vi "main_joystick_test.vi"() -> ()   [LabVIEW 2009]
uses:
  <vilib>/Utility/inputDevices.llb/joystickAcquire.vi
  <vilib>/Utility/inputDevices.llb/closeJoystick.vi
panel:
  out "joystick info":T1(array[cluster]) caption="Angaben zum Joystick"
  out "button 4":bool
  out "button 3":bool
  out "button 2":bool
  out "button 1":bool
  in  "Stopp":bool
  out "error out":errorcluster
  out "Joystick ID":refnum<k1> caption="Geräte-ID"
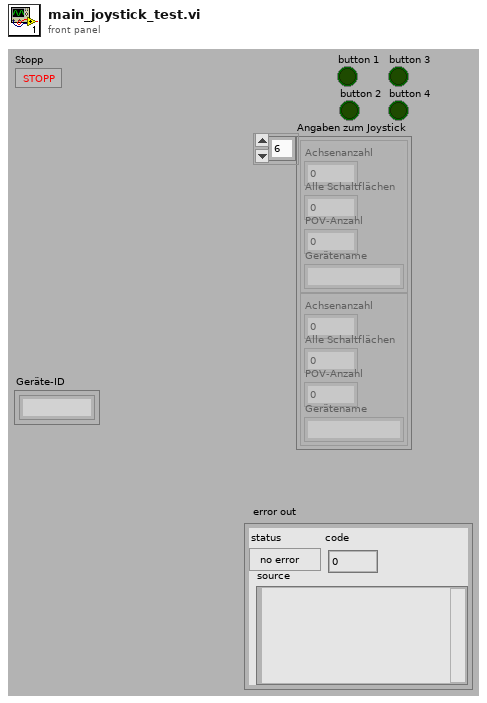
[diagram p1: front panel]
types:
  T1 = cluster{"axes total":u32, "buttons total":u32, "pov total":u32, "device name":string}[]
  T2 = cluster{"X axis":i32, "Y axis":i32, "Z axis":i32, "X axis rotation":i32, "Y axis rotation":i32, "Z axis rotation":i32, "U axis":i32, "V axis":i32}
  T3 = cluster{"button 1":bool, "button 2":bool, "button 3":bool, "button 4":bool, "button 5":bool, "button 6":bool, "button 7":bool, "button 8":bool, "button 9":bool, "button 10":bool, "button 11":bool, "button 12":bool, "button 13":bool, "button 14":bool, "button 15":bool, "button 16":bool, "button 17":bool, "button 18":bool, "button 19":bool, "button 20":bool, "button 21":bool, "button 22":bool, "button 23":bool, "button 24":bool, "button 25":bool, "button 26":bool, "button 27":bool, "button 28":bool, "button 29":bool, "button 30":bool, "button 31":bool, "button 32":bool}
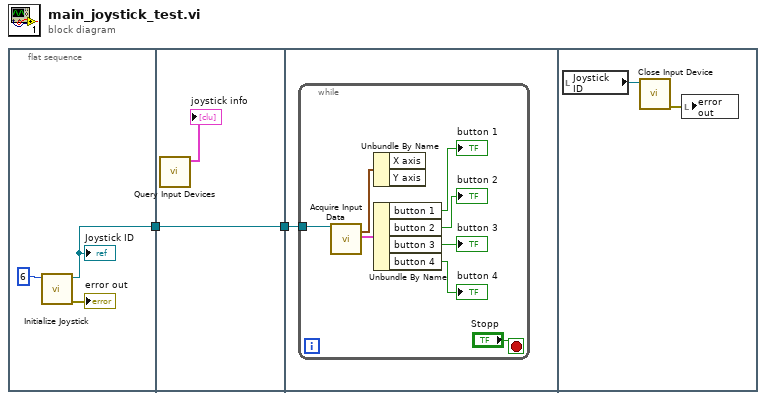
[diagram p0: block diagram]
diagram:
  n1 = flat-sequence {
    tunnel: [w3] -> w2
    tunnel: w2 -> [w7]
    tunnel: [w7] -> w1
    tunnel: w1 -> [w8]
    frame #0 {
      n2 = call <vilib>:"Initialize Joystick.vi"("device index"=6) -> ("error out"=→"error out":errorcluster, "device ID"=w3:refnum<k1>)  [unwired: 9 in]
      "Joystick ID" <- w3
    }
    frame #1 {
      n3 = call <vilib>:"Query Input Devices.vi"() -> ("joystick info"=→"joystick info":T1)  [unwired: 8 in, 3 out]
    }
    frame #2 {
      n4 = while {
        tunnel: w8 -> [w16]
        stop <- "Stopp" stop-if-true
        n5 = call-poly <vilib>:"Acquire Input Data.vi"("device ID"=w16) -> ("axis info"=w14:T2, "button info"=w15:T3)  [unwired: 14 in, 3 out]
        n6 = Unbundle By Name(w14) -> ()  [unwired: 2 out]
        n7 = Unbundle By Name(w15) -> ("button 1"=→"button 1":bool, "button 2"=→"button 2":bool, "button 3"=→"button 3":bool, "button 4"=→"button 4":bool)
      }
    }
    frame #3 {
      n8 = local read "Joystick ID"() -> (w17:refnum<k1>)
      n9 = call-poly <vilib>:"Close Input Device.vi"("device ID"=w17) -> ("error out"=w18:errorcluster)  [unwired: 9 in]
      n10 = local write "error out"(w18) -> ()
    }
  }
